vi "lib Display Relative Time with Days.vi"(10 "seconds":dbl(knob) scale=0.0..1000000.0) -> (1 "HH:MM:SS":string, 2 "Days HH:MM:SS":string)   [LabVIEW 2014]
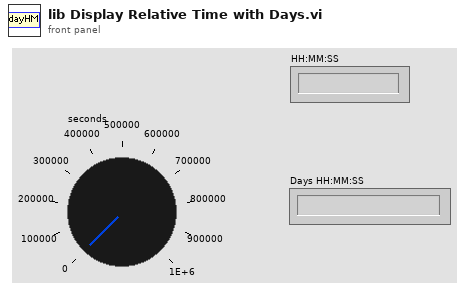
[diagram p1: front panel]
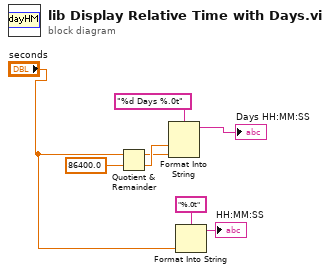
[diagram p0: block diagram]
diagram:
  n1 = Quotient & Remainder(x="seconds", y=86400.0) -> (x-y*floor(x/y)=w4:dbl, floor(x/y)=w5:dbl)
  n2 = Format Into String(format string="%d Days %.0t", w5, w4) -> (resulting string=→"Days HH:MM:SS":string)  [unwired: 2 in, 1 out]
  n3 = Format Into String(format string="%.0t", "seconds") -> (resulting string=→"HH:MM:SS":string)  [unwired: 2 in, 1 out]
